vi "Create Container.vi"(8 "Error In":errorcluster, 11 "Tool Box Builder in":refnum<class "Tool Box Builder.lvclass">) -> (0 "Error Out":errorcluster, 2 "Container":refnum<class "QWidget.lvclass">, 3 "Tool Box Builder out":refnum<class "Tool Box Builder.lvclass">)   [LabVIEW 2014, in "Dynamic GUI Composition and Management.lvlib" / "Tool Box Builder.lvclass"]
doc: "Copyright (c) 2016 Sze Howe Koh\nThis code is licensed under the MIT license"
uses:
  Tool Box Builder.lvclass
  src/LabVIEW/Qt Widgets/QWidget/QWidget.lvclass
  src/LabVIEW/Qt Widgets/QToolBox/QToolBox.lvclass
  Dynamic GUI Composition and Management.lvlib
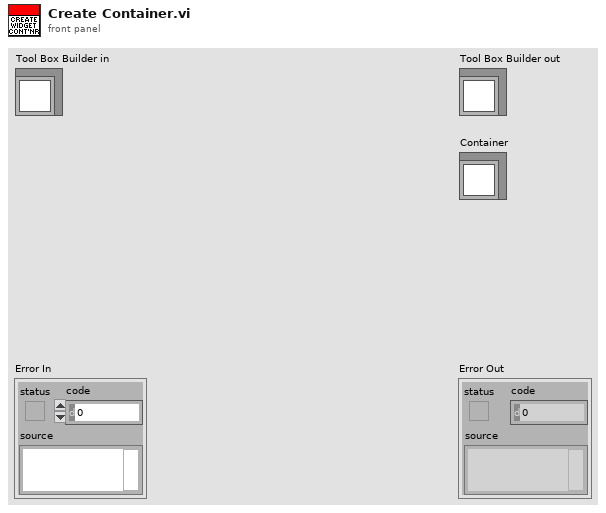
[diagram p1: front panel]
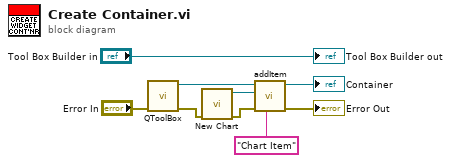
[diagram p0: block diagram]
diagram:
  n1 = call "QToolBox.vi"("Error In"="Error In") -> ("Error Out"=w4:errorcluster, "New QToolBox"=w6:refnum<class "QToolBox.lvclass">)  [unwired: 9 in]
  n2 = call "New Chart.vi"("Error In"=w4) -> ("Error Out"=w3:errorcluster, "New LQChart"=w2:refnum<class "LQChart.lvclass">)  [unwired: 9 in]
  n3 = call "addItem.vi"("text"="Chart Item", "Error In"=w3, "widget"=w2, "QToolBox In"=w6) -> ("Error Out"=→"Error Out":errorcluster, "QToolBox Out"=→"Container":refnum<class "QToolBox.lvclass">)  [unwired: 5 in, 1 out]
  "Tool Box Builder out" <- "Tool Box Builder in"
